vi "Generate DO channel name.vi"(11 "DAQmx Device name":tag) -> (2 "Trigger Term":tag, 3 "Counter Channel":tag)   [LabVIEW 2013]
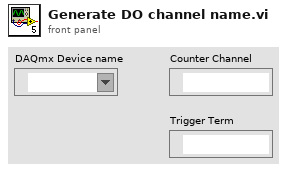
[diagram p1: front panel]
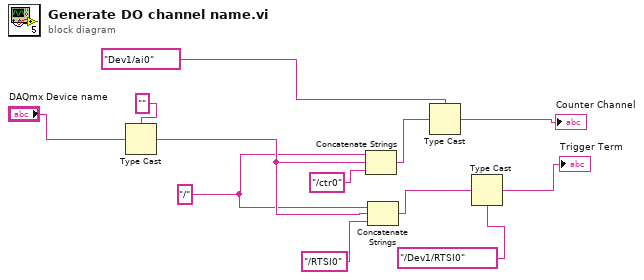
[diagram p0: block diagram]
diagram:
  w1 = "/" ("字符串")
  n1 = Type Cast(type="", x="DAQmx Device name") -> (*(type *) &x=w5:string)
  n2 = Concatenate Strings(w1, w5, "/ctr0" ("字符串")) -> (w8:string)
  n3 = Concatenate Strings(w1, w5, "/RTSI0" ("字符串")) -> (w3:string)
  n4 = Type Cast(type=tag "Dev1/ai0" ("Counter Channel"), x=w8) -> (*(type *) &x=→"Counter Channel":tag)
  n5 = Type Cast(type=tag "/Dev1/RTSI0" ("Trigger Term"), x=w3) -> (*(type *) &x=→"Trigger Term":tag)
